vi "GetDataAndBundle_OP_10.vi"(8 "error in (no error)":errorcluster, 9 "data in":variant[][](array[variant])=[variant, variant, variant, variant, variant, variant, variant, variant, variant, variant, variant, variant, variant, variant, variant, variant, variant, variant], 11 "StaionDataIn":string[](array[string])) -> (0 "error out":errorcluster, 3 "output array":string[](array[string]))   [LabVIEW 2024]
uses:
  <vilib>/addons/database/_DB Variant To Data/Database Variant To Data.xnode
panel:
  out "size(s)":i32
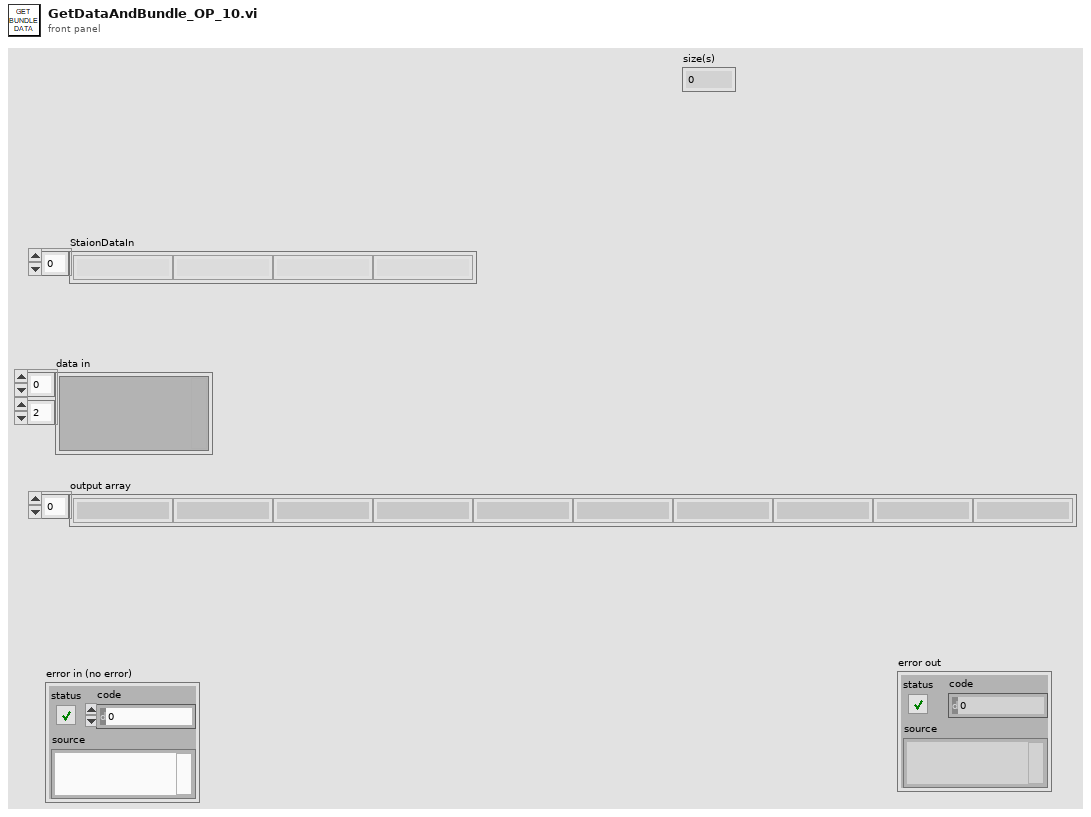
[diagram p1: front panel]
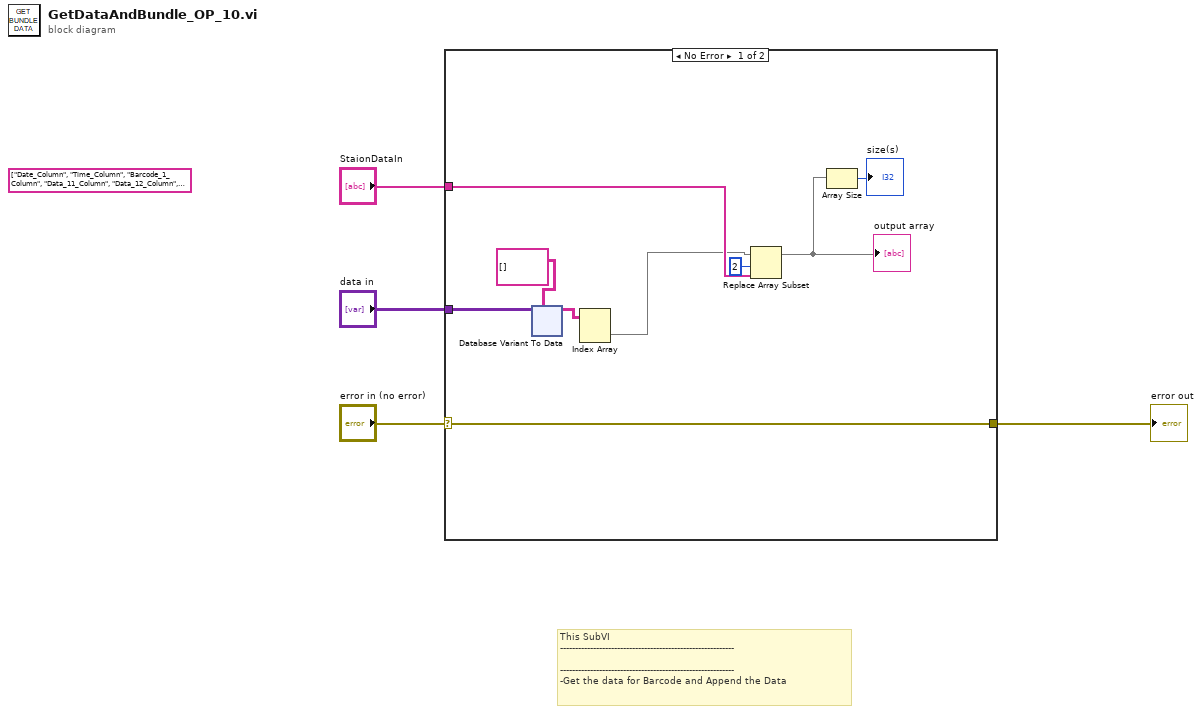
[diagram p0: block diagram]
diagram:
  (unwired) string[] ["Date_Column", "Time_Column", "Barcode_1_Column", "Data_11_Column", "Data_12_Column", "Data_13_Column", "Barcode_2_Column", "Data_21_Column", "Data_22_Column", "Data_23_Column", "Barcode_3_Column", "Data_31_Column", "Data_32_Column", "Data_33_Column", "Barcode_4_Column", "Data_41_Column", "Data_42_Column", "Data_43_Column"] ("appended array")
  # "This SubVI\n----------------------------------------------------------\n\n----------------------------------------------------------\n-Get the data for Barcode and Append the Data"
  n1 = case shown="No Error" "error in (no error)" {
    selector: "error in (no error)" -> [w11 w58]
    tunnel: "data in" -> [w12 _]
    tunnel: [w11 w58] -> w4
    tunnel: "StaionDataIn" -> [w9 _]
    frame No Error {
      n2 = xnode "Database Variant To Data"("database variant"=w12, "type"=string[][] []) -> ("data"=w8:string[][])  [unwired: 1 in, 1 out]
      n3 = Index Array(array=w8) -> (element=w7:string[])  [unwired: 2 in]
      n4 = Replace Array Subset(array=w7, new element=w9, index=2) -> (w6:string[])
      "output array" <- w6
      n5 = Array Size(array=w6) -> (size(s)=→"size(s)":i32)
    }
    frame Error {
    }
  }
  "error out" <- w4
